vi "Get Paths.vi"(8 "error in":errorcluster, 10 "Naming Data":refnum<class "Naming Data.lvclass">, 11 "Namer Decorator in":refnum<class "Namer Decorator.lvclass">) -> (0 "error out":errorcluster, 1 "Received Path":path, 2 "Approved Path":path, 3 "Namer Decorator out":refnum<class "Namer Decorator.lvclass">)   [LabVIEW 2020, in "Approval Tests.lvlib" / "Namer Decorator.lvclass"]
uses:
  Namer Decorator.lvclass
  Naming Data/Naming Data.lvclass
  Namer Decorator.lvclass/Namer Decorator.ctl
  Namer/Namer.lvclass
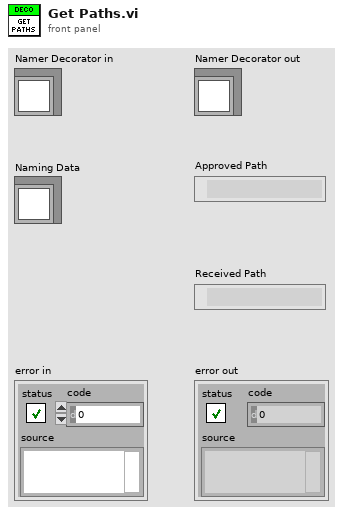
[diagram p1: front panel]
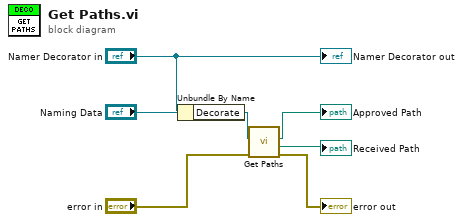
[diagram p0: block diagram]
diagram:
  n1 = Unbundle By Name("Namer Decorator in") -> ("Decorate"=w1:refnum<class "Namer.lvclass">)
  n2 = call-dynamic "Get Paths.vi"("error in"="error in", "Naming Data"="Naming Data", "Namer in"=w1) -> ("error out"=→"error out":errorcluster, "Received Path"=→"Received Path":path, "Approved Path"=→"Approved Path":path)  [unwired: 5 in, 1 out]
  "Namer Decorator out" <- "Namer Decorator in"
